vi "setTime.vi"(0 "connection ID":refnum<k5>, 1 "day":i32, 2 "month":i32, 3 "year":i32, 4 "hour":i32, 5 "error":errorcluster, 6 "minute":i32, 7 "second":i32) -> (14 "connection ID out":refnum<k5>, 19 "error out":errorcluster)   [LabVIEW 2016, in "sen_api.lvlib"]
doc: "Sets system time manually."
uses:
  sen_api.lvlib
panel:
  out "jsonRespIn":string
  out "JSON-response":string="{\"jsonrpc\":\"2.0\",\"method\":\"\",\"params\":[5,1.245,true,\"name\"],\"id\":\"1\"}"
  out "JSON request":string
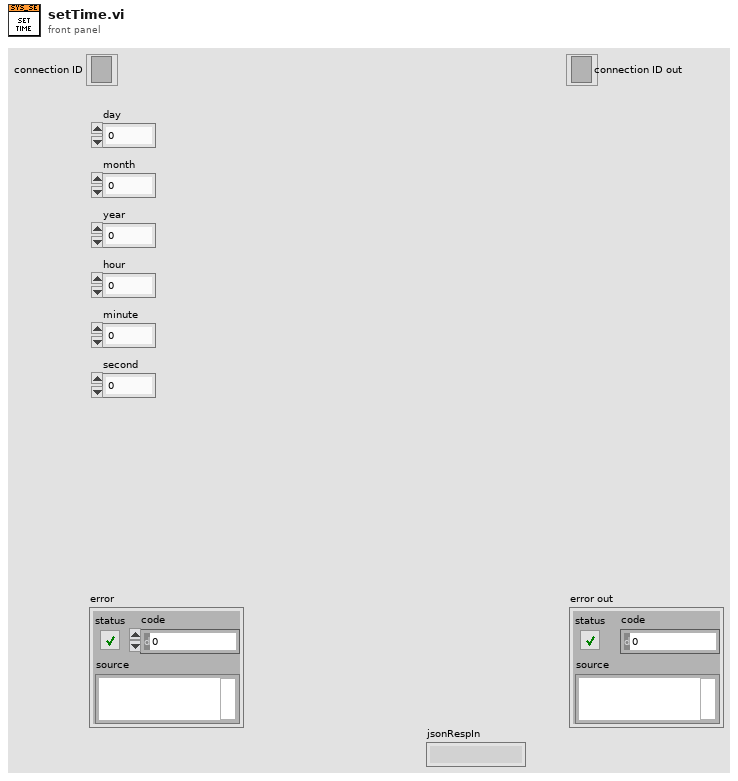
[diagram p1: front panel]
types:
  T1 = cluster{"jsonrpc":string, "method":string, "params":string[], "id":string, "api":i32, "pid":string}
  T2 = enum16{"Standard", "Buffered", "CRLF", "Immediate"}
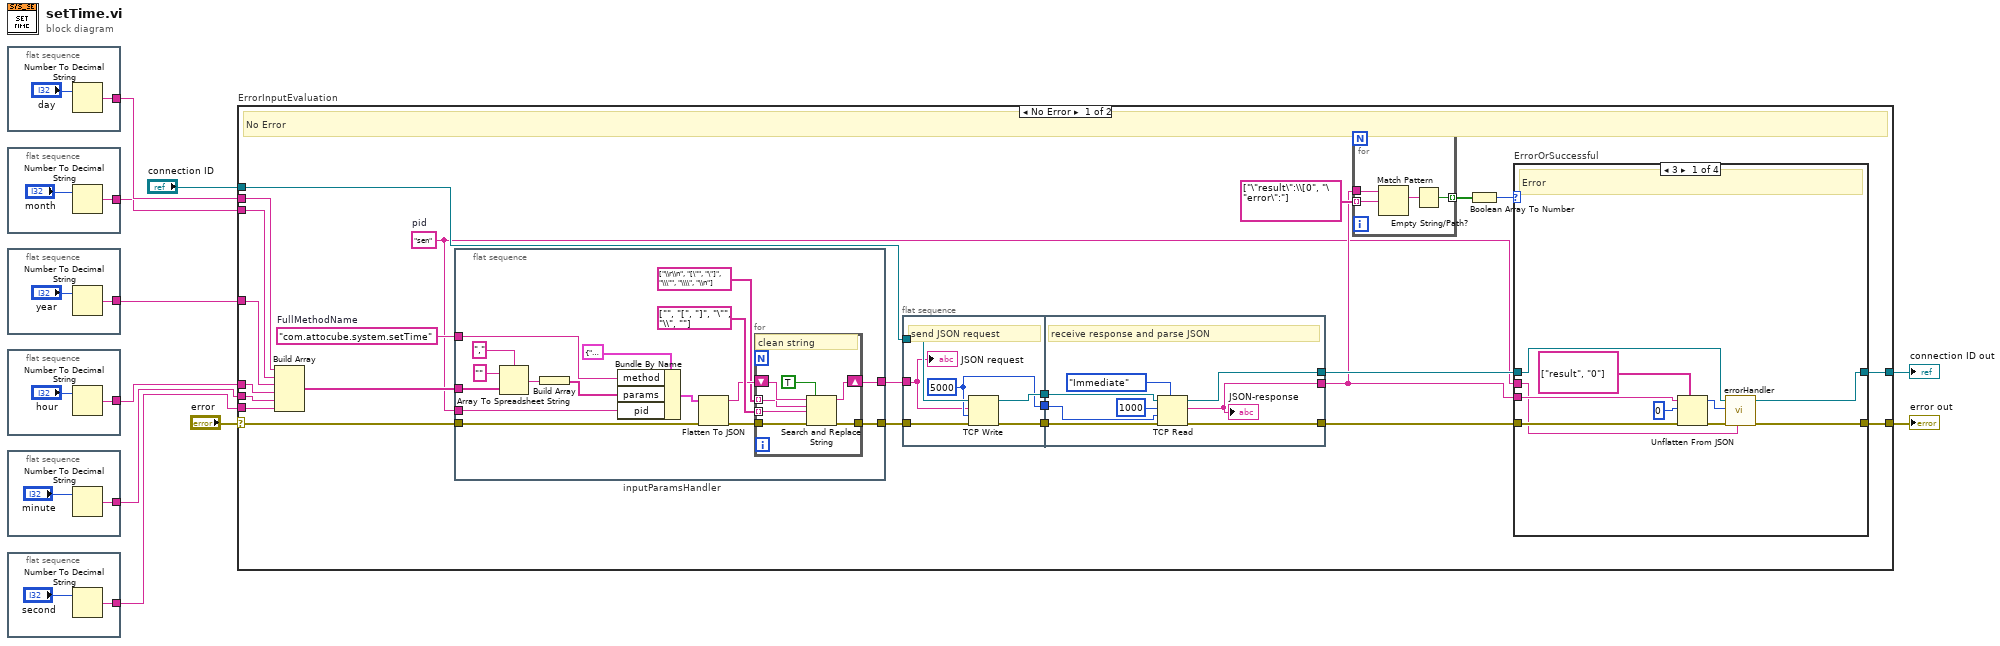
[diagram p0: block diagram]
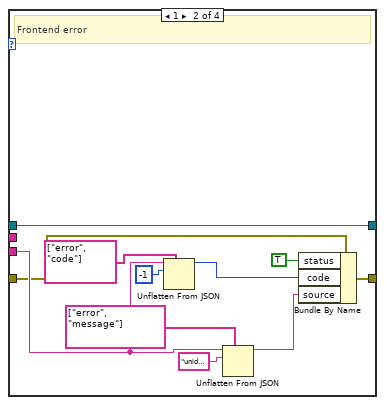
[diagram p2: hidden frame]
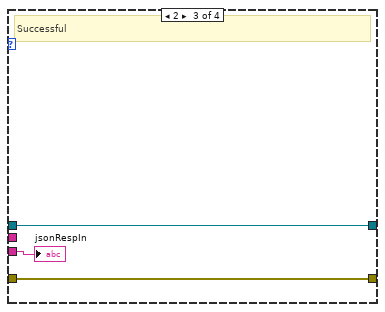
[diagram p3: hidden frame]
diagram:
  n1 = flat-sequence "in_integer" {
    tunnel: [w11] -> w6
    frame #0 {
      n2 = Number To Decimal String(number="day") -> (decimal integer string=w11:string)  [unwired: 1 in]
    }
  }
  n3 = flat-sequence "in_integer" {
    tunnel: [w13] -> w5
    frame #0 {
      n4 = Number To Decimal String(number="month") -> (decimal integer string=w13:string)  [unwired: 1 in]
    }
  }
  n5 = flat-sequence "in_integer" {
    tunnel: [w15] -> w4
    frame #0 {
      n6 = Number To Decimal String(number="year") -> (decimal integer string=w15:string)  [unwired: 1 in]
    }
  }
  n7 = flat-sequence "in_integer" {
    tunnel: [w17] -> w3
    frame #0 {
      n8 = Number To Decimal String(number="hour") -> (decimal integer string=w17:string)  [unwired: 1 in]
    }
  }
  n9 = flat-sequence "in_integer" {
    tunnel: [w19] -> w2
    frame #0 {
      n10 = Number To Decimal String(number="minute") -> (decimal integer string=w19:string)  [unwired: 1 in]
    }
  }
  n11 = flat-sequence "in_integer" {
    tunnel: [w21] -> w1
    frame #0 {
      n12 = Number To Decimal String(number="second") -> (decimal integer string=w21:string)  [unwired: 1 in]
    }
  }
  n13 = case "ErrorInputEvaluation" shown="No Error" "error" {
    selector: "error" -> [w39 w114]
    tunnel: "connection ID" -> [w43 w115]
    tunnel: [w30 w114] -> w9
    tunnel: [w31 w115] -> w8
    tunnel: w6 -> [w28 _]
    tunnel: w5 -> [w27 _]
    tunnel: w4 -> [w26 _]
    tunnel: w3 -> [w25 _]
    tunnel: w2 -> [w24 _]
    tunnel: w1 -> [w23 _]
    frame No Error {
      w29 = "sen"  # pid
      w40 = "com.attocube.system.setTime"  # FullMethodName
      # "No Error"
      n14 = Build Array ("ParametersArrayString")(w28, w27, w26, w25, w24, w23) -> (w38:string[])
      n15 = flat-sequence "inputParamsHandler" {
        tunnel: [w76] -> w37
        tunnel: w38 -> [w83]
        tunnel: w39 -> [w81]
        tunnel: [w78] -> w36
        tunnel: w40 -> [w84]
        tunnel: w29 -> [w73]
        frame #0 {
          n16 = Array To Spreadsheet String(delimiter (Tab)=",", array=w83, 3:"" ("format string")) -> (spreadsheet string=w86:string)
          n17 = Build Array "Build Array"(w86) -> (w82:string[])
          n18 = Bundle By Name(cluster=T1 {"jsonrpc"="2.0", "method"="com.attocube.amc.res.setRESReadOutFreq", "params"=[], "id"="1", "api"=2, "pid"=""} ("Cluster"), "method"=w84, "params"=w82, "pid"=w73) -> (w85:T1)
          n19 = Flatten To JSON(anything=w85, error in (no error)=w81) -> (JSON string=w77:string, 11:w79:errorcluster)  [unwired: 1 in]
          n20 = for {
            tunnel: string[] ["\\r\\n", "[\"", "\"]", "\\\"", "\\\\", "\\n"] ("search string") -> [w92] mode=indexing
            tunnel: string[] ["", "[", "]", "\"", "\\", ""] ("replace string (\"\")") -> [w91] mode=indexing
            shift-right: [w94] -> w76
            shift-left: w77 -> [w93]
            tunnel: w79 -> [w90]
            tunnel: [w89] -> w78
            # "clean string"
            n21 = Search and Replace String(replace all?=TRUE ("replace all? (F)"), input string=w93, search string=w92, replace string=w91, error in=w90) -> (result string=w94:string, error out=w89:errorcluster)  [unwired: 3 in, 2 out]
          }
        }
      }
      n22 = flat-sequence {
        tunnel: w43 -> [w105]
        tunnel: [w103] -> w46
        tunnel: [w104] -> w45
        tunnel: w36 -> [w100]
        tunnel: [w102] -> w44
        tunnel: w37 -> [w101]
        tunnel: [w109] -> w35
        tunnel: w46 -> [w111]
        tunnel: w45 -> [w110]
        tunnel: [w107] -> w34
        tunnel: w44 -> [w108]
        tunnel: [w106] -> w33
        frame #0 {
          w102 = 5000 ("timeout ms (25000)")
          # "send JSON request"
          n23 = TCP Write(connection ID=w105, data in=w101, error in (no error)=w100, 9:w102) -> (connection ID out=w103:refnum<k5>, error out=w104:errorcluster)  [unwired: 1 out]
          "JSON request" <- w101
        }
        frame #1 {
          # "receive response and parse JSON"
          n24 = TCP Read(connection ID=w111, bytes to read=1000, error in (no error)=w110, 7:T2."Immediate" ("mode (standard)"), 9:w108) -> (connection ID out=w109:refnum<k5>, data out=w106:string, error out=w107:errorcluster)
          "JSON-response" <- w106
        }
      }
      n25 = for {
        tunnel: string[] ["\"result\":\\[0", "\"error\":"] ("path") -> [w98] mode=indexing
        tunnel: [w96] -> w41 mode=indexing
        tunnel: w33 -> [w99]
        n26 = Match Pattern(string=w99, regular expression=w98) -> (match substring=w97:string)  [unwired: 1 in, 3 out]
        n27 = Empty String/Path?(string/path=w97) -> (empty?=w96:bool)
      }
      n28 = Boolean Array To Number(Boolean array=w41) -> (number=w32:u32)
      n29 = case "ErrorOrSuccessful" shown="3" w32 {
        tunnel: w33 -> [w50 w59 w68 _]
        tunnel: w35 -> [w54 w57 w70 w72]
        tunnel: [w52 w57 w70 w72] -> w31
        tunnel: [w53 w60 w69 w71] -> w30
        tunnel: w34 -> [w56 w58 w69 w71]
        tunnel: w29 -> [w47 _ _ _]
        frame 3 {
          # "Error"
          n30 = Unflatten From JSON(path=string[] ["result", "0"], JSON string=w50, type and defaults=0, error in (no error)=w56) -> (value=w48:i32, error out=w55:errorcluster)  [unwired: 3 in]
          n31 = call "errorHandler.vi"("pid"=w47, "error in"=w55, "errNbr"=w48, "connection ID"=w54) -> ("error out 2"=w53:errorcluster, "connection ID out"=w52:refnum<k5>)  [unwired: 6 in]
        }
        frame 1 {
          # "Frontend error"
          n32 = Unflatten From JSON(path=string[] ["error", "code"], JSON string=w59, type and defaults=-1) -> (value=w66:i32)  [unwired: 4 in, 1 out]
          n33 = Unflatten From JSON(path=string[] ["error", "message"], JSON string=w59, type and defaults="unidentified error") -> (value=w67:string)  [unwired: 4 in, 1 out]
          n34 = Bundle By Name(cluster=w58, "status"=TRUE, "code"=w66, "source"=w67) -> (w60:errorcluster)
        }
        frame 2 {
          # "Successful"
          "jsonRespIn" <- w68
        }
        frame Default {
          # "NoResponse"
        }
      }
    }
    frame Error {
      # "Error"
    }
  }
  "error out" <- w9
  "connection ID out" <- w8
